vi "LED_control.vi"() -> ()   [LabVIEW 2018]
uses:
  <instrlib>/niDMM/nidmm.llb/niDMM Function.ctl
  <instrlib>/niDMM/nidmm.llb/niDMM Resolution in Digits.ctl
  <instrlib>/niDCPower/nidcpower.llb/niDCPower Measurement Type.ctl
  <vilib>/Instr/_visa.llb/VISA Configure Serial Port (Instr).vi
  <instrlib>/niDMM/nidmm.llb/niDMM Configure Measurement Digits.vi
panel:
  in  "Tab Control":enum32{"Рабочая область", "Служебная область"}(tab)
  out "Тип индикатора":string
  in  "Питание":bool
  in  "Стоп":bool
  in  "Resource Name":refnum<k15>="PXI1Slot2" caption="Первый источник"
  in  "NI DMM 1":refnum<k15>="PXI1Slot3"
  in  "voltlevel_0, V":dbl=6.0 caption="voltage level" format="%_6p"
  in  "curlim_0, A":dbl=0.3 caption="current limit" format="%_6p"
  in  "curlim_2, A":dbl=0.1 caption="current limit" format="%_6p"
  out "currentmes_0, A":dbl caption="measurement" format="%_6g"
  out "currentmes_2, A":dbl caption="measurement" format="%_6g"
  in  "voltlevel_2, V":dbl caption="voltage level" format="%_6p"
  out "chart_2":dbl(graph)=8.556104343922883e-07
  out "chart_0":dbl(graph)=5.42616690347781e-05 caption="Waveform Chart 5"
  in  "curlim_1, A":dbl=0.1 caption="current limit" format="%_6p"
  in  "voltlevel_1, V":dbl=3.0 caption="voltage level" format="%_6p"
  out "chart_1":dbl(graph)=2.456762028615791e-06 caption="Waveform Chart 5"
  out "currentmes_1, A":dbl caption="measurement" format="%_6g"
  in  "NI DMM 1 Current Range 3":string(combo)="-1" caption="Range"
  out "Real Current, А":dbl=1.3612861948786303e-08 format="%.5f"
  in  "NI DMM 1 units 3":string(combo)="1000000" caption="Units"
  out "NI DMM 1 Current Char 3":dbl(graph)=0.013612861948786303
  out "NI DMM 1 Current 3":dbl caption="Current" format="%_6g"
  in  "Arduino":refnum<visa-resource-name>="COM4"
  in  "Сегменты":bool[](array[boolean])=[FALSE, FALSE, FALSE, FALSE, FALSE, FALSE, FALSE, FALSE, FALSE, FALSE]
  in  "Записать":bool
  in  "Command":string="led_on"
  out "Разряд":dbl
  out "+/-":bool
  # "необходимо выдерживать 1 с между нажатиями кнопок"
  # "a"
  # "b"
  # "c"
  # "d"
  # "e"
  # "f"
  # "g"
  # "dp"
  # "all_off - 0\nall_on - 1"
  # "ОЗ: управление сегментами\nкнопки в 0 - горят\nкнопки в 1 - не горят"
  # "ОП: управление сегменатми\nкнопки в 0 - не горят\nкнопки в 1 - горят"
  # "ОЗ - 0\nОП - 1\n(горит)"
  # "прединициализация. Нужно чтобы при запуске \nвсе сегменты+питание инд были либо в 0, либо в 1.\nзатем нужно подключить настоящий индикатор."
  # "Кнопки не горят - 0\nКнопки горят - 1"
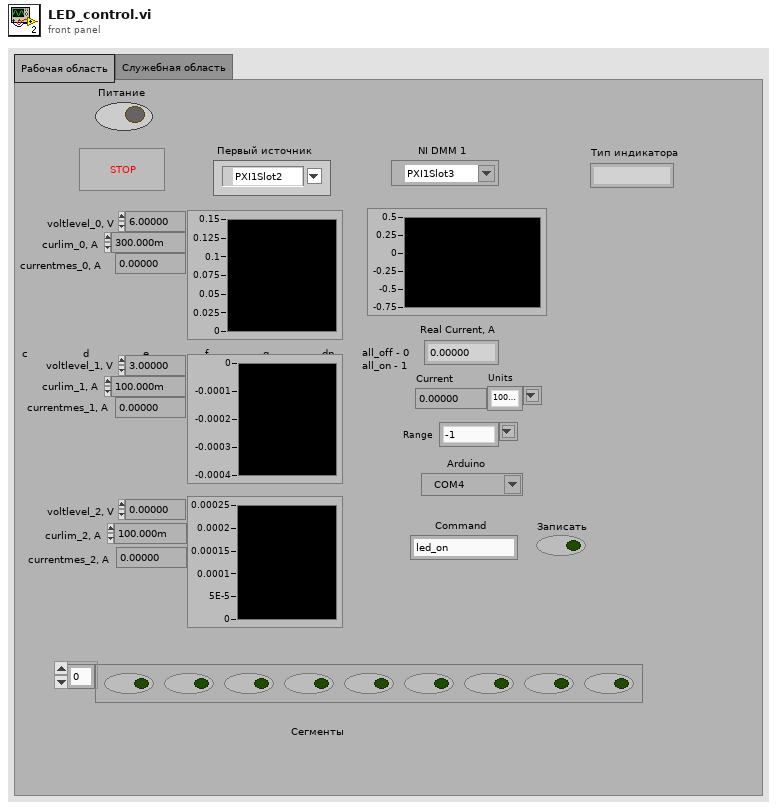
[diagram p1: front panel]
types:
  T1 = typedef "niDMM Function.ctl" = enum16{"DC Volts", "AC Volts", "DC Current", "AC Current", "2-wire Resistance", "4-wire Resistance", "Diode", "Frequency", "Period", "AC Volts DC Coupled", "Capacitance", "Inductance", "Temperature"}
  T2 = typedef "niDMM Resolution in Digits.ctl" = dbl
  T3 = typedef "niDCPower Measurement Type.ctl" = i32
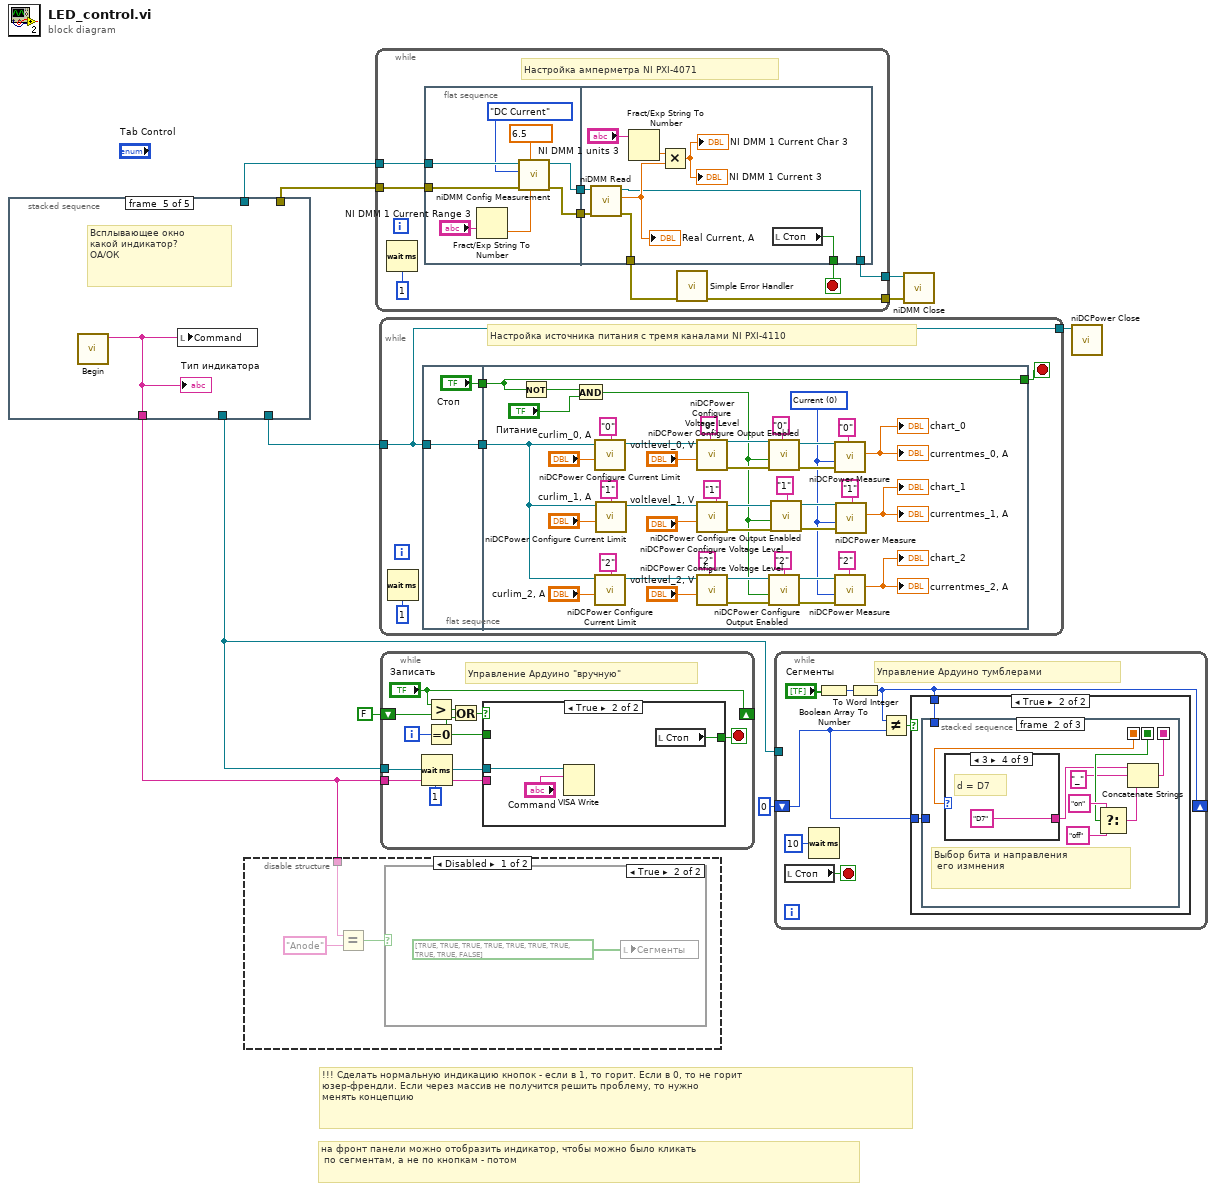
[diagram p0: block diagram]
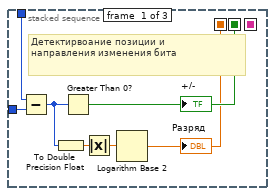
[diagram p5: hidden frame]
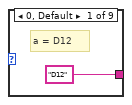
[diagram p6: hidden frame]
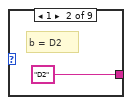
[diagram p7: hidden frame]
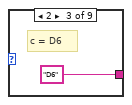
[diagram p8: hidden frame]
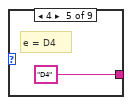
[diagram p9: hidden frame]
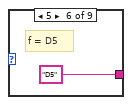
[diagram p10: hidden frame]
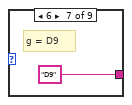
[diagram p11: hidden frame]
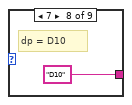
[diagram p12: hidden frame]
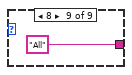
[diagram p13: hidden frame]
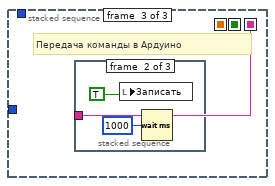
[diagram p14: hidden frame]
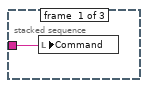
[diagram p15: hidden frame]
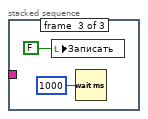
[diagram p16: hidden frame]
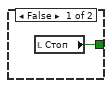
[diagram p17: hidden frame]
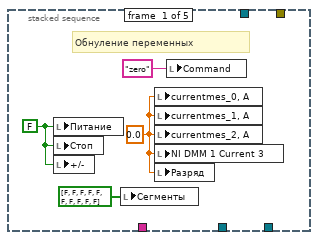
[diagram p18: hidden frame]
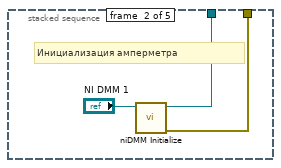
[diagram p19: hidden frame]
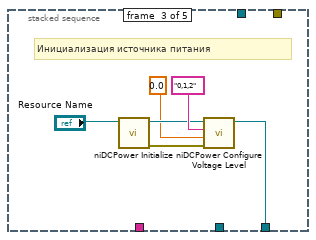
[diagram p20: hidden frame]
diagram:
  # "на фронт панели можно отобразить индикатор, чтобы можно было кликать\n по сегментам, а не по кнопкам - потом"
  # "!!! Сделать нормальную индикацию кнопок - если в 1, то горит. Если в 0, то не горит\nюзер-френдли. Если через массив не получится решить проблему, то нужно\nменять концепцию"
  n1 = stacked-sequence {
    tunnel: [_ _ w20 _ _] -> w7
    tunnel: [_ w16 _ _ _] -> w10
    tunnel: [_ w15 _ _ _] -> w9
    tunnel: [_ _ _ w24 _] -> w4
    tunnel: [_ _ _ _ w27] -> w1
    frame #0 {
      w13 = 0.0 ("currentmes_2")
      w11 = FALSE ("Стоп")
      # "Обнуление переменных"
      n2 = local write "Питание"(w11) -> ()
      n3 = local write "Стоп"(w11) -> ()
      n4 = local write "+/-"(w11) -> ()
      n5 = local write "Сегменты"(bool[] [FALSE, FALSE, FALSE, FALSE, FALSE, FALSE, FALSE, FALSE, FALSE, FALSE] ("Сегменты")) -> ()
      n6 = local write "currentmes_0, A"(w13) -> ()
      n7 = local write "currentmes_1, A"(w13) -> ()
      n8 = local write "currentmes_2, A"(w13) -> ()
      n9 = local write "NI DMM 1 Current 3"(w13) -> ()
      n10 = local write "Разряд"(w13) -> ()
      n11 = local write "Command"("zero" ("Command 2")) -> ()
    }
    frame #1 {
      # "Инициализация амперметра"
      n12 = call <instrlib>:"niDMM Initialize.vi"("Instrument Descriptor"="NI DMM 1") -> ("error out"=w16:errorcluster, "instrument handle out"=w15:refnum<k15>)  [unwired: 9 in]
    }
    frame #2 {
      # "Инициализация источника питания"
      n13 = call <instrlib>:"niDCPower Initialize.vi"("resource name"="Resource Name") -> ("error out"=w19:errorcluster, "instrument handle out"=w21:refnum<k15>)  [unwired: 3 in, 6 out]
      n14 = call <instrlib>:"niDCPower Configure Voltage Level.vi"("error in (no error)"=w19, "voltage level"=0.0, "channel name"="0,1,2", "instrument handle"=w21) -> ("instrument handle out"=w20:refnum<k15>)  [unwired: 6 in, 1 out]
    }
    frame #3 {
      # "Инициализация Ардуино"
      n15 = call-poly "VISA Configure Serial Port"("VISA resource name"="Arduino", "baud rate (9600)"=u32 9600) -> ("VISA resource name out"=w24:refnum<visa-resource-name>)  [unwired: 12 in, 1 out]
    }
    frame #4 {
      # "Всплывающее окно\nкакой индикатор?\nОА/ОК"
      n16 = call "Begin.vi"() -> ("String"=w27:string)  [unwired: 8 in]
      "Тип индикатора" <- w27
      n17 = local write "Command"(w27) -> ()
    }
  }
  n18 = disable-structure shown="Disabled" {
    disable-tunnel: w1 -> [w29 _]
    frame Disabled {
      n19 = Equal?(x=w29, y="Anode") -> (x = y?=w30:bool)
      n20 = case shown="True" w30 {
        frame False {
        }
        frame True {
          n21 = local write "Сегменты"(bool[] [TRUE, TRUE, TRUE, TRUE, TRUE, TRUE, TRUE, TRUE, TRUE, FALSE] ("Сегменты")) -> ()
        }
      }
    }
    frame Enabled {
    }
  }
  n22 = while {
    tunnel: [w38] -> w2
    tunnel: w9 -> [w36]
    tunnel: w10 -> [w35]
    tunnel: [w32] -> w3
    stop <- w34 stop-if-true
    # "Настройка амперметра NI PXI-4071"
    n23 = Wait (ms)(milliseconds to wait=u32 1) -> ()  [unwired: 1 out]
    n24 = flat-sequence {
      tunnel: [w45] -> w40
      tunnel: w36 -> [w43]
      tunnel: w35 -> [w47]
      tunnel: [w44] -> w39
      tunnel: w40 -> [w53]
      tunnel: w39 -> [w56]
      tunnel: [w51] -> w34
      tunnel: [w50] -> w32
      tunnel: [w49] -> w33
      frame #0 {
        w41 = T2 6.5 items=["3 1/2"=3.5, "4 1/2"=4.5, "5 1/2"=5.5, "6 1/2"=6.5, "7 1/2"=7.5] ("Resolution in Digits")
        n25 = Fract/Exp String To Number(string="NI DMM 1 Current Range 3") -> (number=w46:dbl)  [unwired: 3 in, 1 out]
        n26 = call-poly <instrlib>:"niDMM Config Measurement.vi"("Range"=w46, "Resolution in Digits"=w41, "error in (no error)"=w47, "Function"=niDMM_Function."DC Current" ("Measurement Type"), "instrument handle"=w43) -> ("error out"=w44:errorcluster, "instrument handle out"=w45:refnum<k15>)  [unwired: 5 in]
      }
      frame #1 {
        n27 = call <instrlib>:"niDMM Read.vi"("error in (no error)"=w56, "instrument handle"=w53) -> ("error out"=w49:errorcluster, "Measurement"=w52:dbl, "instrument handle out"=w50:refnum<k15>)  [unwired: 7 in]
        "Real Current, А" <- w52
        n28 = Fract/Exp String To Number(string="NI DMM 1 units 3") -> (number=w54:dbl)  [unwired: 3 in, 1 out]
        n29 = Multiply(x=w54, y=w52) -> (x*y=→"NI DMM 1 Current 3" →"NI DMM 1 Current Char 3":dbl)
        n30 = local read "Стоп"() -> (w51:bool)
      }
    }
    n31 = call <vilib>:"Simple Error Handler.vi"("error in (no error)"=w33) -> ("error out"=w38:errorcluster)  [unwired: 1 in, 7 out]
  }
  n32 = while {
    tunnel: w7 -> [w58]
    tunnel: [w58] -> w6
    stop <- w59 stop-if-true
    # "Настройка источника питания с тремя каналами NI PXI-4110"
    n33 = Wait (ms)(milliseconds to wait=u32 1) -> ()  [unwired: 1 out]
    n34 = flat-sequence {
      tunnel: w58 -> [w64]
      tunnel: [w64] -> w61
      tunnel: ["Стоп"] -> w60
      tunnel: w61 -> [w72]
      tunnel: w60 -> [w106]
      tunnel: [w106] -> w59
      frame #0 {
      }
      frame #1 {
        w71 = T3 0 items=["Current", "Voltage"] ("measurement type")
        n35 = Not(x=w106) -> (.not. x?=w105:bool)
        n36 = And(x=w105, y="Питание") -> (x .and. y?=w67:bool)
        n37 = call <instrlib>:"niDCPower Configure Current Limit.vi"("current limit"="curlim_0, A", "channel name"="0", "instrument handle"=w72) -> ("instrument handle out"=w91:refnum<k15>)  [unwired: 7 in, 1 out]
        n38 = call <instrlib>:"niDCPower Configure Current Limit.vi"("current limit"="curlim_2, A", "channel name"="2", "instrument handle"=w72) -> ("instrument handle out"=w90:refnum<k15>)  [unwired: 7 in, 1 out]
        n39 = call <instrlib>:"niDCPower Configure Current Limit.vi"("current limit"="curlim_1, A", "channel name"="1", "instrument handle"=w72) -> ("instrument handle out"=w99:refnum<k15>)  [unwired: 7 in, 1 out]
        n40 = call <instrlib>:"niDCPower Configure Voltage Level.vi"("voltage level"="voltlevel_0, V", "channel name"="0", "instrument handle"=w91) -> ("error out"=w96:errorcluster, "instrument handle out"=w93:refnum<k15>)  [unwired: 7 in]
        n41 = call <instrlib>:"niDCPower Configure Voltage Level.vi"("voltage level"="voltlevel_1, V", "channel name"="1", "instrument handle"=w99) -> ("error out"=w102:errorcluster, "instrument handle out"=w100:refnum<k15>)  [unwired: 7 in]
        n42 = call <instrlib>:"niDCPower Configure Voltage Level.vi"("voltage level"="voltlevel_2, V", "channel name"="2", "instrument handle"=w90) -> ("error out"=w95:errorcluster, "instrument handle out"=w94:refnum<k15>)  [unwired: 7 in]
        n43 = call <instrlib>:"niDCPower Configure Output Enabled.vi"("error in (no error)"=w96, "output enabled"=w67, "channel name"="0", "instrument handle"=w93) -> ("error out"=w86:errorcluster, "instrument handle out"=w87:refnum<k15>)  [unwired: 6 in]
        n44 = call <instrlib>:"niDCPower Configure Output Enabled.vi"("error in (no error)"=w95, "output enabled"=w67, "channel name"="2", "instrument handle"=w94) -> ("error out"=w85:errorcluster, "instrument handle out"=w84:refnum<k15>)  [unwired: 6 in]
        n45 = call <instrlib>:"niDCPower Configure Output Enabled.vi"("error in (no error)"=w102, "output enabled"=w67, "channel name"="1", "instrument handle"=w100) -> ("error out"=w103:errorcluster, "instrument handle out"=w101:refnum<k15>)  [unwired: 6 in]
        n46 = call <instrlib>:"niDCPower Measure.vi"("error in (no error)"=w86, "measurement type"=w71, "channel name"="0", "instrument handle"=w87) -> ("measurement"=→"currentmes_0, A" →"chart_0":dbl)  [unwired: 5 in, 2 out]
        n47 = call <instrlib>:"niDCPower Measure.vi"("error in (no error)"=w85, "measurement type"=w71, "channel name"="2", "instrument handle"=w84) -> ("measurement"=→"currentmes_2, A" →"chart_2":dbl)  [unwired: 5 in, 2 out]
        n48 = call <instrlib>:"niDCPower Measure.vi"("error in (no error)"=w103, "measurement type"=w71, "channel name"="1", "instrument handle"=w101) -> ("measurement"=→"chart_1" →"currentmes_1, A":dbl)  [unwired: 5 in, 2 out]
      }
    }
  }
  n49 = while {
    tunnel: w4 -> [w112]
    shift-right: ["Записать"] -> _
    shift-left: FALSE ("Записать") -> [w114]
    tunnel: w1 -> [w110]
    i -> [w111]
    stop <- w115 stop-if-true
    # "Управление Ардуино \"вручную\""
    n50 = Wait (ms)(milliseconds to wait=u32 1) -> ()  [unwired: 1 out]
    n51 = Greater?(x="Записать", y=w114) -> (0:w108:bool)
    n52 = Equal To 0?(x=w111) -> (x = 0?=w107:bool)
    n53 = Or(x=w108, y=w107) -> (x .or. y?=w109:bool)
    n54 = case shown="True" w109 {
      tunnel: w112 -> [_ w120]
      tunnel: [w117 w119] -> w115
      tunnel: w110 -> [_ _]
      tunnel: w107 -> [_ _]
      frame False {
        n55 = local read "Стоп"() -> (w117:bool)
      }
      frame True {
        n56 = VISA Write(VISA resource name=w120, write buffer="Command") -> ()  [unwired: 1 in, 3 out]
        n57 = local read "Стоп"() -> (w119:bool)
      }
    }
  }
  n58 = while {
    shift-right: [w121] -> _
    shift-left: i16 0 -> [w123]
    tunnel: w4 -> [_]
    stop <- w127 stop-if-true
    # "Управление Ардуино тумблерами"
    n59 = local read "Стоп"() -> (w127:bool)
    n60 = Wait (ms)(milliseconds to wait=u32 10 ("millisecond timer value")) -> ()  [unwired: 1 out]
    n61 = Boolean Array To Number(Boolean array="Сегменты") -> (number=w122:u32)
    n62 = To Word Integer(number=w122) -> (16bit integer=w121:i16)
    n63 = Not Equal?(x=w121, y=w123) -> (x != y?=w124:bool)
    n64 = case shown="True" w124 {
      tunnel: w121 -> [_ w128]
      tunnel: w123 -> [_ w129]
      frame False {
      }
      frame True {
        n65 = stacked-sequence {
          seq-local: [w132 _ _] -> [_ w142 _]
          seq-local: [w130 _ _] -> [_ w137 _]
          seq-local: [_ w138 _] -> [_ _ w154]
          tunnel: w128 -> [w134 _ _]
          tunnel: w129 -> [w133 _ _]
          frame #0 {
            # "Детектирвоание позиции и\nнаправления изменения бита"
            n66 = Subtract(x=w134, y=w133) -> (x-y=w135:i16)
            n67 = To Double Precision Float(number=w135) -> (double precision float=w136:dbl)
            n68 = Greater Than 0?(x=w135) -> (x > 0?=w132:bool)
            "+/-" <- w132
            n69 = Absolute Value(x=w136) -> (abs(x)=w131:dbl)
            n70 = Logarithm Base 2(1:w131) -> (0:w130:dbl)
            "Разряд" <- w130
          }
          frame #1 {
            # "Выбор бита и направления\n его измнения"
            n71 = case shown="3" w137 {
              tunnel: ["D12" "D2" "D6" "D7" "D4" "D5" "D9" "D10" "All"] -> w140
              frame 0, Default {
                # "a = D12"
              }
              frame 1 {
                # "b = D2"
              }
              frame 2 {
                # "c = D6"
              }
              frame 3 {
                # "d = D7"
              }
              frame 4 {
                # "e = D4"
              }
              frame 5 {
                # "f = D5"
              }
              frame 6 {
                # "g = D9"
              }
              frame 7 {
                # "dp = D10"
              }
              frame 8 {
              }
            }
            n72 = Select(t="on", s=w142, f="off") -> (s? t:f=w139:string)
            n73 = Concatenate Strings(w140, "_" ("string"), w139) -> (w138:string)
          }
          frame #2 {
            # "Передача команды в Ардуино"
            n74 = stacked-sequence {
              tunnel: w154 -> [w155 _ _]
              frame #0 {
                n75 = local write "Command"(w155) -> ()
              }
              frame #1 {
                n76 = local write "Записать"(TRUE ("Записать")) -> ()
                n77 = Wait (ms)(milliseconds to wait=u32 1000) -> ()  [unwired: 1 out]
              }
              frame #2 {
                n78 = local write "Записать"(FALSE ("Записать")) -> ()
                n79 = Wait (ms)(milliseconds to wait=u32 1000) -> ()  [unwired: 1 out]
              }
            }
          }
        }
      }
    }
  }
  n80 = call <instrlib>:"niDMM Close.vi"("error in (no error)"=w2, "instrument handle"=w3) -> ()  [unwired: 9 in, 1 out]
  n81 = call <instrlib>:"niDCPower Close.vi"("instrument handle"=w6) -> ()  [unwired: 10 in, 1 out]
